vi "KHE - Default Directorys.vi"(8 "error in (no error)":errorcluster, 11 "Directory":enum16{"Root", "Config", "Results"}(ring)) -> (0 "error out":errorcluster, 3 "Path Out":path)   [LabVIEW 2016]
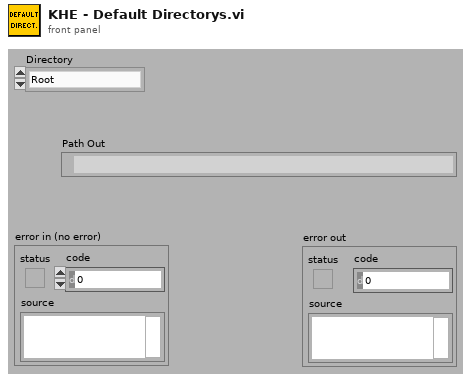
[diagram p1: front panel]
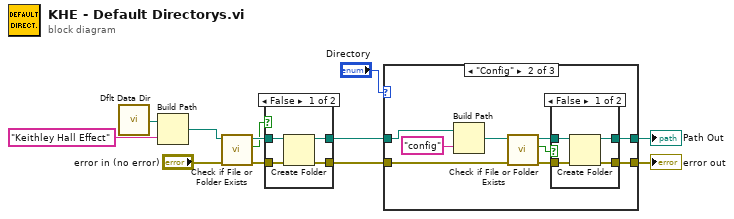
[diagram p0: block diagram]
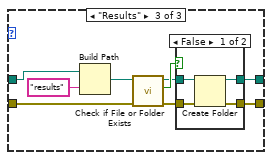
[diagram p4: hidden frame]
diagram:
  n1 = call <vilib>:"Dflt Data Dir.vi"() -> ("App:Default Data Directory"=w7:path)
  n2 = Build Path(base path=w7, name or relative path="Keithley Hall Effect") -> (appended path=w9:path)
  n3 = call <vilib>:"Check if File or Folder Exists.vi"("error in (no error)"="error in (no error)", "path"=w9) -> ("error out"=w12:errorcluster, "file or folder exists?"=w10:bool, "dup path"=w11:path)  [unwired: 7 out]
  n4 = case shown="False" w10 {
    tunnel: w11 -> [w16 w18]
    tunnel: w12 -> [w15 w17]
    tunnel: [w14 w18] -> w5
    tunnel: [w13 w17] -> w4
    frame False {
      n5 = Create Folder(path (use dialog)=w16, error in=w15) -> (created path=w14:path, error out=w13:errorcluster)  [unwired: 2 out]
    }
    frame True {
    }
  }
  n6 = case shown="\"Config\"" "Directory" {
    tunnel: w5 -> [w20 w29 w44]
    tunnel: w4 -> [w19 w26 w41]
    tunnel: [w20 w22 w37] -> w2
    tunnel: [w19 w21 w36] -> w1
    frame "Root", Default {
    }
    frame "Config" {
      n7 = Build Path(base path=w29, name or relative path="config") -> (appended path=w27:path)
      n8 = call <vilib>:"Check if File or Folder Exists.vi"("error in (no error)"=w26, "path"=w27) -> ("error out"=w24:errorcluster, "file or folder exists?"=w25:bool, "dup path"=w23:path)  [unwired: 7 out]
      n9 = case shown="False" w25 {
        tunnel: w24 -> [w33 w34]
        tunnel: w23 -> [w32 w35]
        tunnel: [w31 w35] -> w22
        tunnel: [w30 w34] -> w21
        frame False {
          n10 = Create Folder(path (use dialog)=w32, error in=w33) -> (created path=w31:path, error out=w30:errorcluster)  [unwired: 2 out]
        }
        frame True {
        }
      }
    }
    frame "Results" {
      n11 = Build Path(base path=w44, name or relative path="results") -> (appended path=w42:path)
      n12 = call <vilib>:"Check if File or Folder Exists.vi"("error in (no error)"=w41, "path"=w42) -> ("error out"=w39:errorcluster, "file or folder exists?"=w40:bool, "dup path"=w38:path)  [unwired: 7 out]
      n13 = case shown="False" w40 {
        tunnel: w39 -> [w48 w49]
        tunnel: w38 -> [w47 w50]
        tunnel: [w46 w50] -> w37
        tunnel: [w45 w49] -> w36
        frame False {
          n14 = Create Folder(path (use dialog)=w47, error in=w48) -> (created path=w46:path, error out=w45:errorcluster)  [unwired: 2 out]
        }
        frame True {
        }
      }
    }
  }
  "Path Out" <- w2
  "error out" <- w1
